vi "Laser 1 Operations L3.vi"(8 "Error in":errorcluster caption="Error in (no error)", 11 "UI elements cluster":T2) -> (0 "Error out":errorcluster)   [LabVIEW 2020]
uses:
  Typedefs/UI ctrl refs cluster.ctl
  Typedefs/Laser control knob.ctl
  Typedefs/Frame Size.ctl
  Typedefs/Plane Mode.ctl
  Typedefs/PMT control knob.ctl
  Typedefs/XY Stage_Move.ctl
  Typedefs/test_fpga_control.ctl
  Acquisition/Typedefs/Ref DAQ Param.ctl
  User Interface/Misc/Experiment Type.ctl
  User Interface/Misc/Biology Information.ctl
  Type Defs/Ls1 Operations.ctl
  Typedefs/HW config states enum.ctl
  Type Defs/Ls1 User Ops.ctl
  Serial Comms/Visa resource.ctl
  Typedefs/fgv_actions.ctl
  Global Variables/General Globals.vi
  Global Variables/gl_UI Ctrl Refs.vi
panel:
  out "Laser Ops  actions":T1
  out "Loop itr":i32
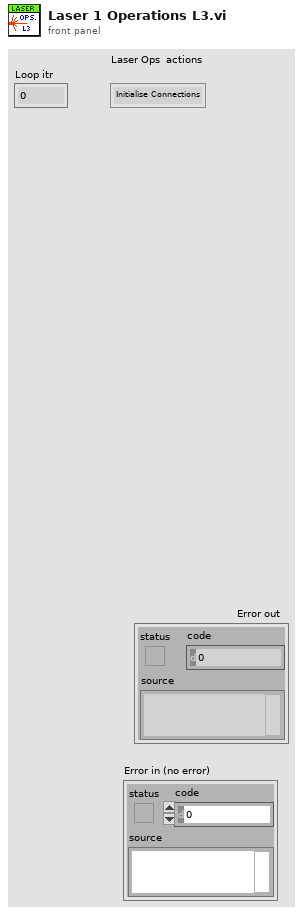
[diagram p1: front panel]
types:
  T1 = typedef "Ls1 Operations.ctl" = enum16{"Initialise Connections", "Initialise system", "Check Status", "Open/Close Shutter", "Start/Stop Pump Peak Hold", "Set wavelength", "Close"}
  T2 = typedef "UI ctrl refs cluster.ctl" = cluster{"Top level VI path":path, "Top level VI ref":refnum<vi>, "User menu ref":refnum<k9>, "Sub Panel control":refnum<vi>, "Imaging Param Tab":refnum<vi>, "Occurrence-Start drivers":refnum<k4>, "Occurrence-Speed logging initialised":refnum<k4>, "Occurrence-XYZ stage initialised":refnum<k4>, "Exit button":refnum<vi>, "Status ind":refnum<vi>, "Set as origin":refnum<vi>, "Speed Logging":refnum<vi>, "Time Lapse":refnum<vi>, "Live Imaging":refnum<vi>, "AOL Z Stack":refnum<vi>, "Motor Z Stack":refnum<vi>, "Funct Acq button":refnum<vi>, "Hard Shutter":refnum<vi>, "Virtual Shutter":refnum<vi>, "Laser Power":refnum<vi>, "AOL Mode":refnum<vi>, "Frame Size":refnum<vi>, "Field of View":refnum<vi>, "Dwell Time":refnum<vi>, "Zoom":refnum<vi>, "AOL Z":refnum<vi>, "Objective":refnum<vi>, "Axis":refnum<vi>, "Paths & Names":refnum<vi>, "Experiment folder path (ind.)":refnum<vi>, "Last State (Ind.)":refnum<vi>, "Averages":refnum<vi>, "Angle (degrees)":refnum<vi>, "X centre":refnum<vi>, "Y centre":refnum<vi>, "Plane Mode":refnum<vi>, "# Planes":refnum<vi>, "Z Start":refnum<vi>, "Z Stop":refnum<vi>, "Z Step":refnum<vi>, "PMT 1":refnum<vi>, "PMT 2":refnum<vi>, "Stage XYZ Position":refnum<vi>, "Pockels@Z Start":refnum<vi>, "Pockels@Z Stop":refnum<vi>, "Obtain Z Start":refnum<vi>, "Obtain Z Stop":refnum<vi>, "Live stim.trig.period":refnum<vi>, "Live stim.trig.enable":refnum<vi>, "Movement Correction":refnum<vi>, "Load Reference Image":refnum<vi>, "XY Stage Move":refnum<vi>, "MovCor Cluster":refnum<vi>, "RefDAQParam":refnum<vi>, "Funct. Acq. Pockels Modulation":refnum<vi>, "Ref Laser Power":refnum<vi>, "Enable Video Recording":refnum<vi>, "Video Record-Live Imaging":refnum<vi>, "Video Record-Funct acq":refnum<vi>, "Reference Source":refnum<vi>, "AOL Z-stack Chirps Ready (ind)":refnum<vi>, "Target time between mov.cor. ref triggers (ms)":refnum<vi>, "Funct. Acq. Ref frame save":refnum<vi>, "Tracking button":refnum<vi>, "Show ref plots window":refnum<vi>, "Center freq ind (nm)":refnum<vi>, "Pickup mode (ind)":refnum<vi>, "Logging queue (ind)":refnum<vi>, "Back aperture power (ind.)":refnum<vi>, "Power after objective (ind.)":refnum<vi>, "Switch user":refnum<vi>, "Ls1 Conn. Status":refnum<vi>, "Ls1Tuning Status":refnum<vi>, "Ls1 Faults":refnum<vi>, "Ls1 Connection":refnum<vi>, "Ls1 Mode":refnum<vi>, "Ls1 POWER [mW]":refnum<vi>, "Ls1Shutter":refnum<vi>, "Ls1 Wavelength":refnum<vi>, "Ls1 Note":refnum<vi>, "Ls1 Confirm Wav":refnum<vi>, "Ls1 PreChrp Prism1":refnum<vi>, "Ls1 PreChrp Prism2":refnum<vi>, "Ls1 wav top Ind":refnum<vi>, "Ls1 power top Ind":refnum<vi>, "Ls1 Pump peak Hold":refnum<vi>, "Ls1 Status Ind":refnum<vi>, "Ls1 wav cancel":refnum<vi>, "Experiment Type":refnum<vi>, "Biology Information":refnum<vi>, "Camera recording status":refnum<vi>, "Optimise Obj. Pos.":refnum<vi>}
  T3 = typedef "Ls1 User Ops.ctl" = enum16{"Setup", "Initialise", "Disable Controls", "Enable Controls", "Update Connection Info", "Update Laser Warning", "Update Laser status", "Update Laser status - sel", "Update Laser Wav.", "Update Laser Power", "Update prechiper settings", "Update Laser Note", "Update Shutter Status", "Close"}
  T4 = typedef "HW config states enum.ctl" = enum16{"Load from file", "Save to file", "Save backup", "Write all", "Read all", "Write XY stage settings", "Write DAQ FPGA settings", "Write Control FPGA settings", "Write Phys Channels", "Write System Config", "Write HW Config", "Save System Config", "Save HW Config", "Clear", "Compare from file"}
  T5 = typedef "Visa resource.ctl" = cluster{"VISA resource name":refnum<visa-resource-name>, "baud rate":u32}
  T6 = typedef "fgv_actions.ctl" = enum16{"Get", "Set"}
  T7 = typedef "System Configuration.ctl" = cluster{"Laser wavelength (nm)":dbl, "DAQ FPGA System":T8, "Control system":T9}
  T8 = typedef "DAQ FPGA system config.ctl" = cluster{"Clock Freq (MHz) ":dbl, "Samples Wait after Trigger":u16, "AOD fill":u16, "StartupDelay":i32, "Slip Cycle (clock cycles)":u32, "Add Cycle":bool}
  T9 = typedef "CTRL system config.ctl" = cluster{"AOD 1 Amplitude":i16, "AOD 2 Amplitude":i16, "AOD 3 Amplitude":i16, "AOD 4 Amplitude":i16, "AOD 5 Amplitude":i16, "AOD 6 Amplitude":i16, "T0 (ns)":dbl, "Ta (ns)":dbl, "Data Time Interval (ns)":dbl, "Ctrl FPGA Clock (MHz)":dbl}
  T10 = typedef "Hardware Configuration settings.ctl" = cluster{"Dev. PC":bool, "Swap XY on stage":bool, "No of AOD":u8, "MC Supported":bool, "Axial MC":bool, "Computer MAC address":string, "Externalise Triggers":bool, "Trigger HW config":T11, "DAQmx Chan":T12, "XYZ Stage Control Config":T13, "XY stage available":bool, "XY Comms Config Cluster":T14, "Y stage available":bool, "Y Comms Config Cluster":T14, "Z stage available":bool, "Z Comms Config Cluster ":T14, "Encoder available":bool, "Encoder":T16, "VidRec available":bool, "Cam VidRec":T17, "Laser Power Control HW config":T18, "Laser 1 available":bool, "Laser 1 config cluster":T19, "Prechirper 1 available":bool, "Prechirper 1 config cluster":T20, "Control system.FPGA available?":bool, "Control Sys. HW config":T21, "DAQ FPGA HW Config":T22, "PMT Control Voltage Limits":T26}
  T11 = typedef "Triggers HW config.ctl" = cluster{"Available Device List":i32, "Device Address":string}
  T12 = typedef "DAQmx physical channels cluster.ctl" = cluster{"Pockels AO":tag, "Hard shutter AO":tag, "PMT AOs":tag, "Galvo AOs":tag, "Power meter AI":tag}
  T13 = typedef "XYZControlConfig.ctl" = enum16{"None", "XYZ", "XY-Z", "X-Y-Z", "Z"}
  T14 = typedef "Peripherals comms config cluster.ctl" = cluster{"Name":string, "Device Address":string, "Port ":u16, "Baudrate":i32, "Comms Type":T15}
  T15 = typedef "Comms Type.ctl" = enum16{"GPIB-IEEE488", "Serial-RS232", "Serial-RS485", "Serial-RS422", "Serial-USB", "Ethernet-TCP/IP", "Ethernet-UDP"}
  T16 = typedef "Encoder config cluster.ctl" = cluster{"IP address":string, "Port":u16, "Wheel radius (cm)":dbl, "Encoder Trigger":tag}
  T17 = typedef "Cam VidRec HW config setup cluster.ctl" = cluster{"DO flag-Video record":tag, "DO flag-Trial start":tag}
  T18 = typedef "Laser Power Control HW config.ctl" = cluster{"Laser Power Control":string, "Laser Power Modulation Control":enum16{"NI", "FPGA"}}
  T19 = typedef "Laser 1 config cluster.ctl" = cluster{"COM port":refnum<visa-resource-name>, "Baud Rate":i32, "Type":string}
  T20 = typedef "PreChirper 1 config cluster.ctl" = cluster{"Type":string, "Baud Rate":i32, "COM port":refnum<visa-resource-name>}
  T21 = typedef "Control Sys HW config cluster.ctl" = cluster{"Control system.FPGA Type":enum16{"Virtex 5", "Virtex 7"}, "Control system.Network adapter name":string, "Control system.MAC address":string, "Control system.Ethernet Port":u32, "Control system.Ethernet Port Opened":bool}
  T22 = typedef "DAQ FPGA HW config cluster.ctl" = cluster{"FGPA Ref":T23, "Target":T24, "input card type":T25}
  T23 = typedef "FPGA Ref.ctl" = refnum<k20>
  T24 = typedef "nirio_resource_hc.ctl" = tag
  T25 = typedef "FPGA input type AC-DC.ctl" = enum16{"AC Card", "DC Card"}
  T26 = typedef "PMT Control Voltage limits.ctl" = cluster{"Lower Limit":dbl, "Upper Limit":dbl}
  T27 = typedef "AOL_Globals.ctl" = cluster{"Imaging Protocol":T28, "Number of POI":u16, "Number of Miniscans":u16, "Number of Trials":u16, "Number of Cycles ":u64, "# Averaged Frames":u16, "Laser power (%)":u8, "Pockels (V)":dbl, "Acquisition Length (sec)":dbl, "Fill time (us)":dbl, "POI Dwell time (us)":dbl, "Miniscan Dwell time per pixel (us)":dbl, "PMT 1":dbl, "PMT 2":dbl, "Back Apperture (mA)":dbl, "Frame Size":T29, "Center Frequency":dbl, "Field of View (um)":dbl, "Field of View (norm)":dbl, "DwellTime (us)":dbl, "Ref Dwell Time (us)":dbl, "Wavelength (nm)":dbl, "Zoom":dbl, "AOL Z":dbl, "AOL Mode":T30, "GridXY":dbl, "GridZ":dbl, "TriggerPeriod (sec)":dbl, "Number of Pixels in Miniscan":u16, "Experiment folder path":path, "X centre":dbl, "Y centre":dbl, "Angle (degrees)":dbl, "Angle Xs (degrees)":dbl, "Angle Ys (degrees)":dbl, "Plane Mode":T31, "Threshold":u16[], "Regenerate Chirps":bool, "Rectangle ROI length (pixels)":u16, "Rectangle ROI height (pixels)":u16, "AOD fill":u16, "StartupDelay":i32, "Samples Wait after Trigger":u16, "Slip Cycle":u32, "Add Cycle":bool, "Functional Mode":T32, "Z Start":dbl, "Z Stop":dbl, "# Planes":i32, "Total Pixels":i32, "Variable Miniscan Pixels":u16[], "Use Variable Length":bool, "Use Variable Resolution":bool, "Laser power (%) at Z Start":u8, "Laser power (%) at Z Stop":u8, "Ref Z Step":i8}
  T28 = typedef "Imaging Protocols enum.ctl" = enum16{"AOL Z-Stack", "Motor Z Stack", "Parameter Sweep", "Functional Acquisition", "Single Plane Acquisition", "Volume Acquisition", "Live Imaging", "Live Plane Imaging", "Live Volume Imaging"}
  T29 = typedef "Frame Size.ctl" = u16
  T30 = typedef "AOL modes.ctl" = enum16{"Raster", "Structural", "Pointing", "Mini Scan", "Alignment"}
  T31 = typedef "Plane Mode.ctl" = u16
  T32 = typedef "Functional Mode.ctl" = enum16{"Point", "Line", "Patch", "Plane", "Volume"}
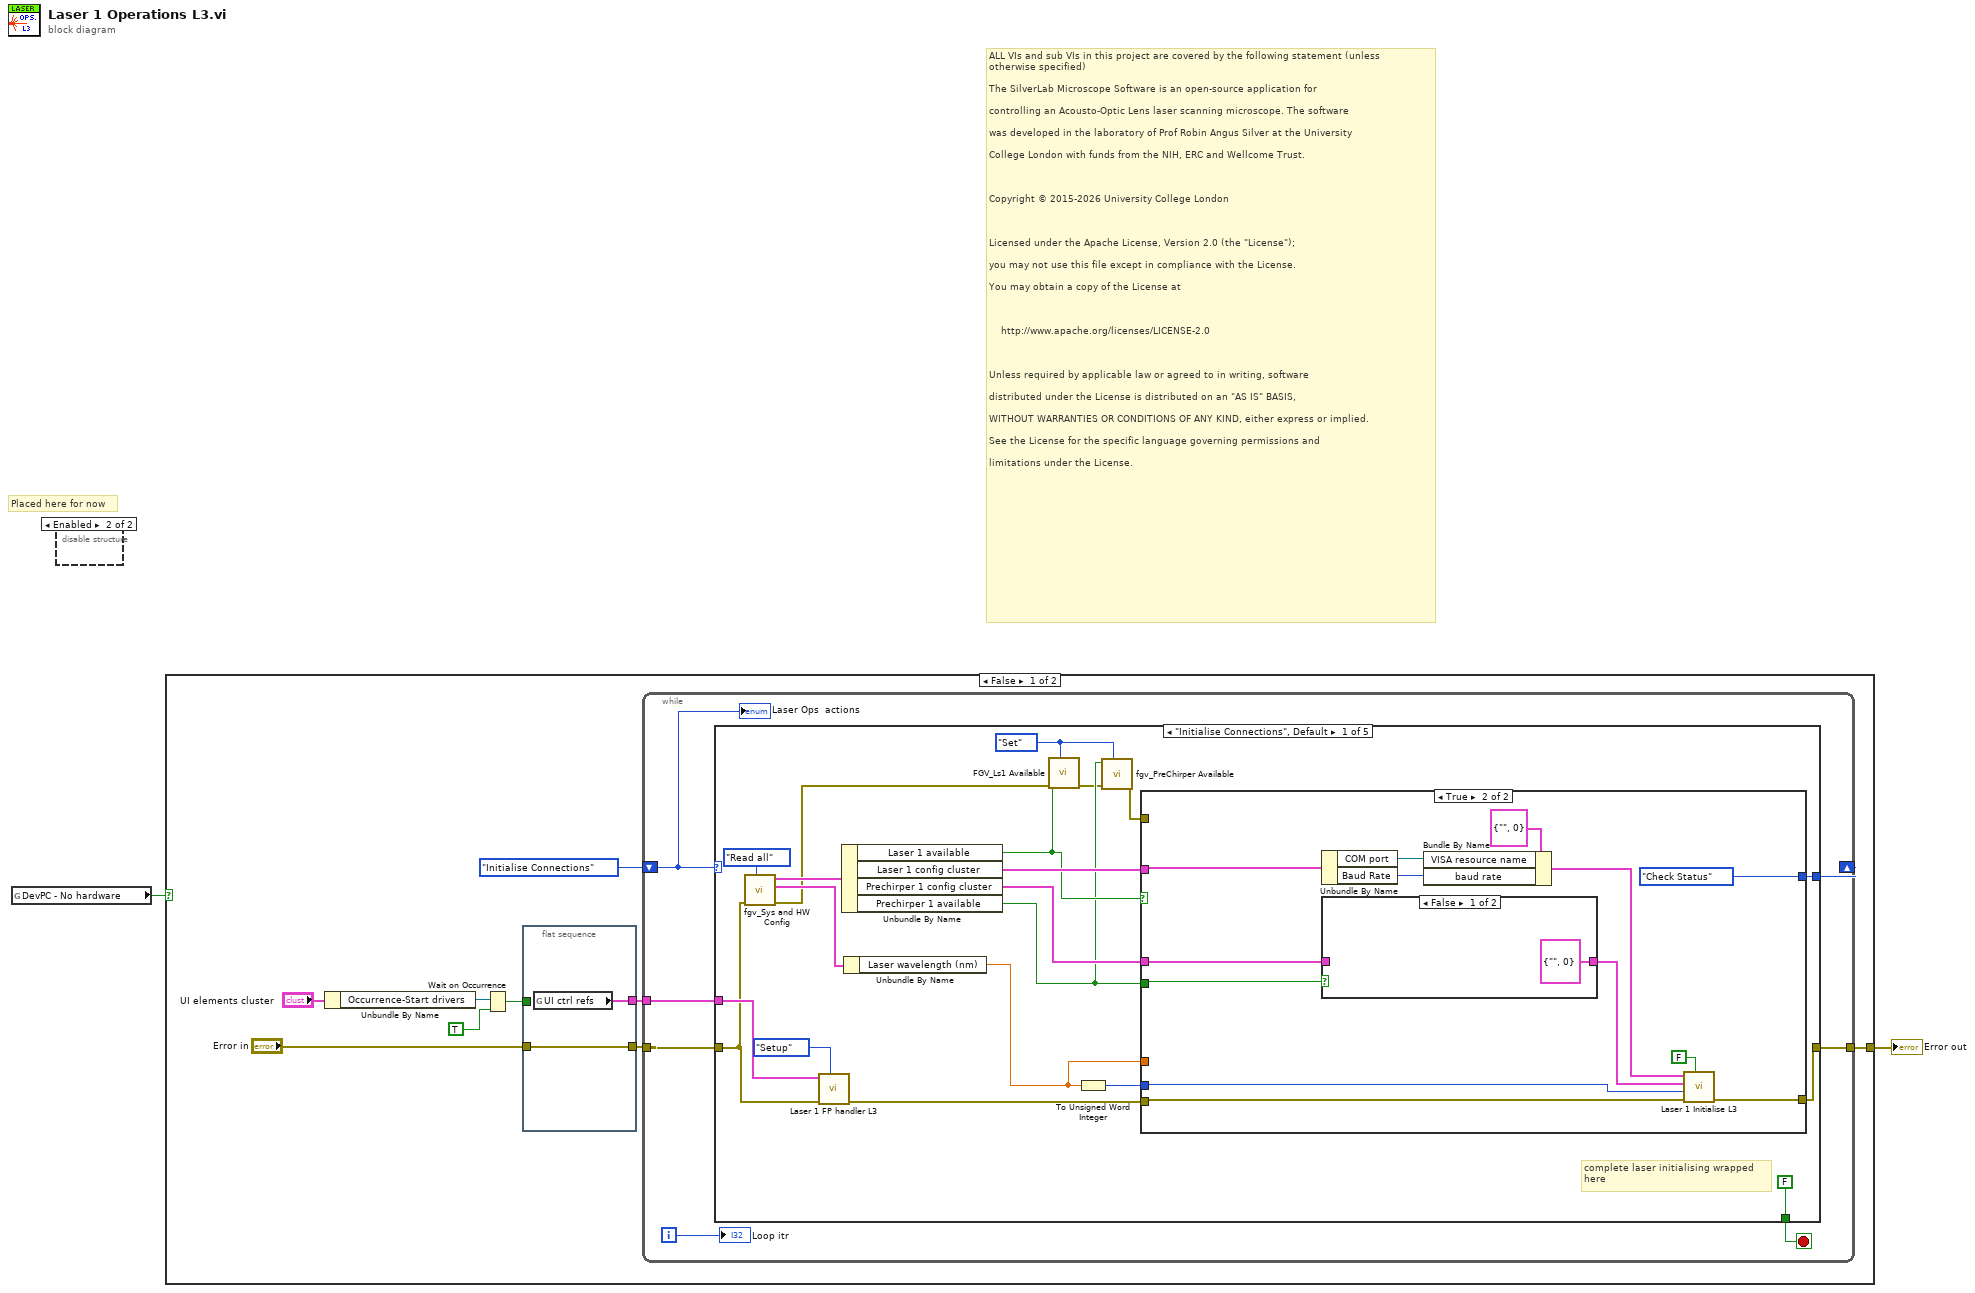
[diagram p0: block diagram]
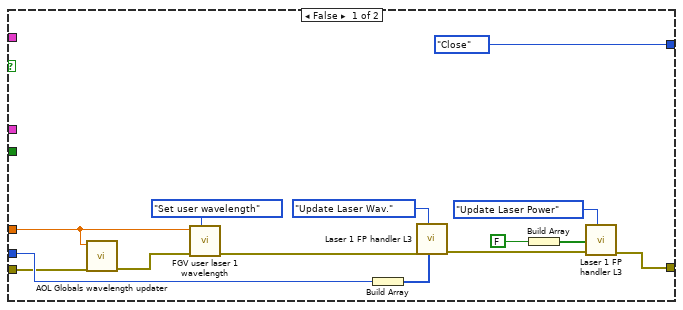
[diagram p2: hidden frame]
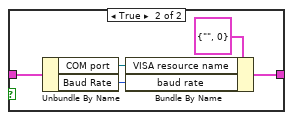
[diagram p3: hidden frame]
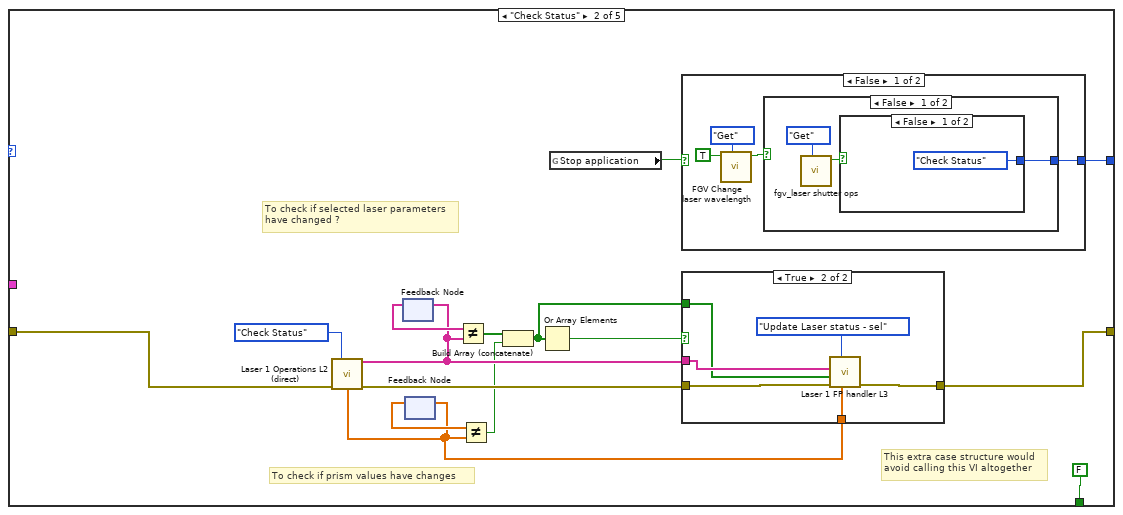
[diagram p4: hidden frame]
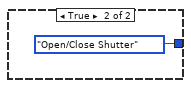
[diagram p5: hidden frame]
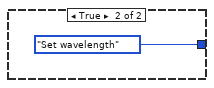
[diagram p6: hidden frame]
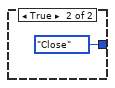
[diagram p7: hidden frame]
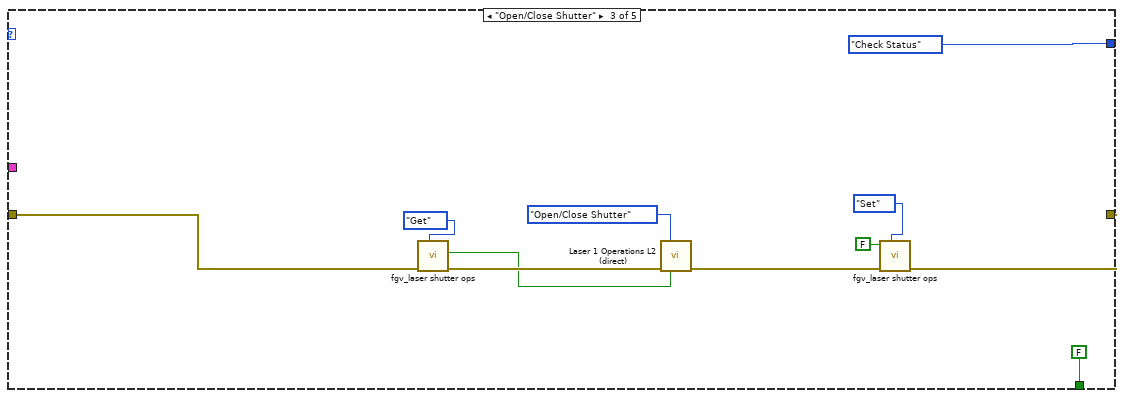
[diagram p9: hidden frame]
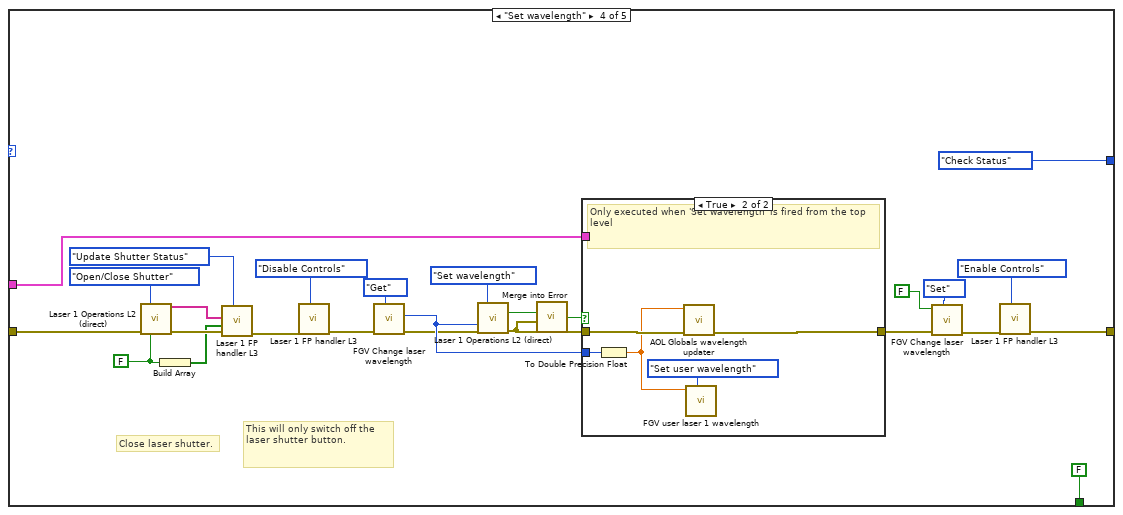
[diagram p10: hidden frame]
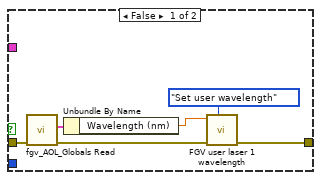
[diagram p11: hidden frame]
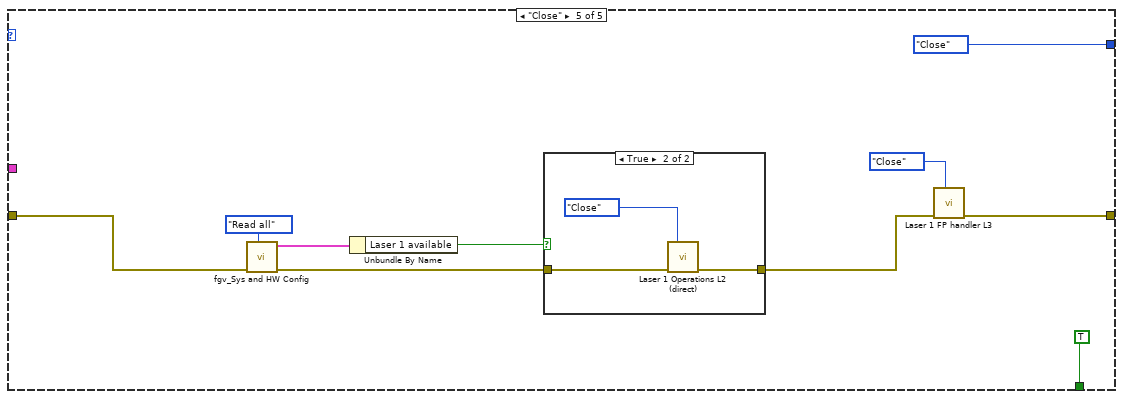
[diagram p12: hidden frame]
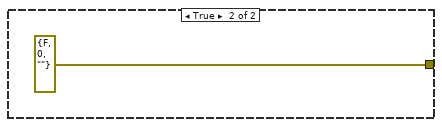
[diagram p14: hidden frame]
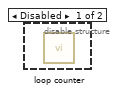
[diagram p15: hidden frame]
diagram:
  # "ALL VIs and sub VIs in this project are covered by the following statement (unless \notherwise specified)\n\nThe SilverLab Microscope Software is an open-source application for\n\ncontrolling an Acousto-Optic Lens laser scanning microscope. The software\n\nwas developed in the laboratory of Prof Robin Angus Silver at the University\n\nCollege London with funds from the NIH, ERC and Wellcome Trust.\n\n \n\nCopyright © 2015-2026 University College London\n\n \n\nLicensed under the Apache License, Version 2.0 (the \"License\");\n\nyou may not use this file except in compliance with the License.\n\nYou may obtain a copy of the License at\n\n \n\n    http://www.apache.org/licenses/LICENSE-2.0\n\n \n\nUnless required by applicable law or agreed to in writing, software\n\ndistributed under the License is distributed on an \"AS IS\" BASIS,\n\nWITHOUT WARRANTIES OR CONDITIONS OF ANY KIND, either express or implied.\n\nSee the License for the specific language governing permissions and\n\nlimitations under the License."
  # "Placed here for now"
  n1 = global read "General Globals.vi" "DevPC - No hardware"() -> (w1:bool)
  n2 = disable-structure shown="Enabled" {
    frame Disabled {
      n3 = call "loop counter.vi"() -> ()  [unwired: 9 in, 1 out]
    }
    frame Enabled {
    }
  }
  n4 = case shown="False" w1 {
    tunnel: [w11 errorcluster {"status"=FALSE, "code"=0, "source"=""} ("error out")] -> w2
    frame False {
      n5 = Unbundle By Name("UI elements cluster") -> ("Occurrence-Start drivers"=w6:refnum<k4>)
      n6 = Wait on Occurrence(1:TRUE ("ignore previous (T)"), 2:w6) -> (0:w5:bool)  [unwired: 1 in]
      n7 = flat-sequence {
        tunnel: w5 -> [_]
        tunnel: "Error in" -> [w13]
        tunnel: [w13] -> w9
        tunnel: [w12] -> w3
        frame #0 {
          n8 = global read "gl_UI Ctrl Refs.vi" "UI ctrl refs"() -> (w12:T2)
        }
      }
      n9 = while {
        tunnel: w9 -> [w20]
        tunnel: w3 -> [w19]
        shift-right: [w16] -> _
        shift-left: Ls1_Operations."Initialise Connections" ("Laser Ops\n actions") -> [w17]
        tunnel: [w18] -> w11
        i -> [w14]
        stop <- w15 stop-if-true
        n10 = case shown="\"Initialise Connections\", Default" w17 {
          tunnel: w20 -> [w24 w88 w113 w130 w161]
          tunnel: w19 -> [w40 _ _ w139 _]
          tunnel: [w39 w83 w107 w119 w155] -> w18
          tunnel: [w34 w81 Ls1_Operations."Check Status" ("Laser Ops\n actions") Ls1_Operations."Check Status" ("Laser Ops\n actions") Ls1_Operations."Close" ("Laser Ops\n actions")] -> w16
          tunnel: [FALSE FALSE FALSE FALSE TRUE] -> w15
          frame "Initialise Connections", Default {
            w30 = enum16{"Get", "Set"}."Set" ("FGV Actions")
            # "complete laser initialising wrapped \nhere"
            n11 = call "fgv_Sys and HW Config.vi"("Function"=HW_config_states_enum."Read all", "error in (no error)"=w24) -> ("error out"=w23:errorcluster, "System Config OUT"=w27:T7, "Hardware Configuration OUT"=w28:T10)  [unwired: 7 in]
            n12 = call "Laser 1 FP handler L3.vi"("FP Ops"=Ls1_User_Ops."Setup", "Error in"=w24, "UI elements cluster"=w40) -> ("Error out"=w26:errorcluster)  [unwired: 6 in, 2 out]
            n13 = Unbundle By Name(w28) -> ("Laser 1 available"=w31:bool, "Laser 1 config cluster"=w38:T19, "Prechirper 1 config cluster"=w37:T20, "Prechirper 1 available"=w29:bool)
            n14 = Unbundle By Name(w27) -> ("Laser wavelength (nm)"=w25:dbl)
            n15 = call "FGV_Ls1 Available.vi"("FGV Actions"=w30, "error in (no error)"=w23, "Laser Available ? IN"=w31) -> ("error out"=w22:errorcluster)  [unwired: 7 in, 1 out]
            n16 = To Unsigned Word Integer(number=w25) -> (unsigned 16bit integer=w35:u16)
            n17 = call "fgv_PreChirper Available.vi"("FGV Actions"=w30, "error in (no error)"=w22, "PreChirper Available ? IN"=w29) -> ("error out"=w21:errorcluster)  [unwired: 7 in, 1 out]
            n18 = case shown="True" w31 {
              tunnel: [w44 w67] -> w39
              tunnel: w38 -> [_ w63]
              tunnel: w37 -> [_ w62]
              tunnel: w26 -> [w43 w61]
              tunnel: w35 -> [w52 w60]
              tunnel: [Ls1_Operations."Close" ("Laser Ops\n actions") Ls1_Operations."Check Status" ("Laser Ops\n actions")] -> w34
              tunnel: w25 -> [w41 _]
              tunnel: w29 -> [_ w55]
              tunnel: w21 -> [_ _]
              frame False {
                n19 = call "AOL Globals wavelength updater.vi"("error in (no error)"=w43, "Laser wavelength (nm)"=w41) -> ("error out"=w42:errorcluster)  [unwired: 9 in]
                n20 = call "FGV user laser 1 wavelength.vi"("FGV Actions"=enum16{"Get", "Set user wavelength"}."Set user wavelength", "error in (no error)"=w42, "Laser wavelength IN"=w41) -> ("error out"=w45:errorcluster)  [unwired: 7 in, 1 out]
                n21 = Build Array(w52) -> (w51:u16[])
                n22 = call "Laser 1 FP handler L3.vi"("Numeric"=w51, "FP Ops"=Ls1_User_Ops."Update Laser Wav.", "Error in"=w45) -> ("Error out"=w50:errorcluster)  [unwired: 6 in, 2 out]
                n23 = Build Array(FALSE) -> (w47:bool[])
                n24 = call "Laser 1 FP handler L3.vi"("FP Ops"=Ls1_User_Ops."Update Laser Power", "Error in"=w50, "Boolean"=w47) -> ("Error out"=w44:errorcluster)  [unwired: 6 in, 2 out]
              }
              frame True {
                n25 = Unbundle By Name(w63) -> ("COM port"=w58:refnum<visa-resource-name>, "Baud Rate"=w57:i32)
                n26 = case shown="False" w55 {
                  tunnel: [T5 {"VISA resource name"="", "baud rate"=0} ("Ls1 Visa \nresource") w73] -> w64
                  tunnel: w62 -> [_ w72]
                  frame False {
                  }
                  frame True {
                    n27 = Unbundle By Name(w72) -> ("COM port"=w70:refnum<visa-resource-name>, "Baud Rate"=w69:i32)
                    n28 = Bundle By Name(cluster=T5 {"VISA resource name"="", "baud rate"=0} ("Ls1 Visa \nresource"), "VISA resource name"=w70, "baud rate"=w69) -> (w73:T5)
                  }
                }
                n29 = Bundle By Name(cluster=T5 {"VISA resource name"="", "baud rate"=0} ("Ls1 Visa \nresource"), "VISA resource name"=w58, "baud rate"=w57) -> (w65:T5)
                n30 = call "Laser 1 Initialise L3.vi"("Independent?"=FALSE ("from FGV ?"), "Error in"=w61, "Wavelength (set) [nm]"=w60, "PreChrp1 \nVisa resource"=w64, "Ls1 Visa \nresource"=w65) -> ("Error out"=w67:errorcluster)  [unwired: 6 in]
              }
            }
          }
          frame "Check Status" {
            # "This extra case structure would\navoid calling this VI altogether"
            # "To check if prism values have changes"
            # "To check if selected laser parameters\nhave changed ?"
            n31 = call "Laser 1 Operations L2 (direct).vi"("Laser Ops\n actions"=Ls1_Operations."Check Status" ("Laser Ops\n actions"), "error in (no error)"=w88) -> ("Ls Data"=w82:string[], "prism Values"=w74:dbl[], "error out"=w84:errorcluster)  [unwired: 8 in, 3 out]
            n32 = feedback-in #1(w82) -> ()
            n33 = feedback #1() -> (w85:string[])  [unwired: 1 in]
            n34 = feedback #2() -> (w78:dbl[])  [unwired: 1 in]
            n35 = feedback-in #2(w74) -> ()
            n36 = Not Equal?(x=w85, y=w82) -> (x != y?=w77:bool[])
            n37 = Not Equal?(x=w78, y=w74) -> (x != y?=w76:bool)
            n38 = Build Array (concatenate)(w77, w76) -> (w75:bool[])
            n39 = Or Array Elements(Boolean array=w75) -> (logical OR=w79:bool)
            n40 = global read "General Globals.vi" "Stop application"() -> (w80:bool)
            n41 = case shown="False" w80 {
              tunnel: [w89 Ls1_Operations."Close" ("Laser Ops\n actions")] -> w81
              frame False {
                n42 = call "FGV Change laser wavelength.vi"("FGV Actions"=enum16{"Get", "Set"}."Get", "Change Wavelength ? IN"=TRUE) -> ("Change Wavelength ? OUT"=w90:bool)  [unwired: 7 in, 2 out]
                n43 = case shown="False" w90 {
                  tunnel: [w93 Ls1_Operations."Set wavelength" ("Laser Ops\n actions")] -> w89
                  frame False {
                    n44 = call "fgv_laser shutter ops.vi"("FGV Actions"=fgv_actions."Get") -> ("Operate Shutter [OUT}"=w94:bool)  [unwired: 8 in, 2 out]
                    n45 = case shown="False" w94 {
                      tunnel: [Ls1_Operations."Check Status" ("Laser Ops\n actions") Ls1_Operations."Open/Close Shutter" ("Laser Ops\n actions")] -> w93
                      frame False {
                      }
                      frame True {
                      }
                    }
                  }
                  frame True {
                  }
                }
              }
              frame True {
              }
            }
            n46 = case shown="True" w79 {
              tunnel: w84 -> [w100 w106]
              tunnel: [w100 w105] -> w83
              tunnel: w82 -> [_ w103]
              tunnel: w75 -> [_ w102]
              tunnel: w74 -> [_ w101]
              frame False {
              }
              frame True {
                n47 = call "Laser 1 FP handler L3.vi"("Numeric"=w101, "FP Ops"=Ls1_User_Ops."Update Laser status - sel", "Error in"=w106, "Boolean"=w102, "I/p string(s)"=w103) -> ("Error out"=w105:errorcluster)  [unwired: 4 in, 2 out]
              }
            }
          }
          frame "Open/Close Shutter" {
            n48 = call "fgv_laser shutter ops.vi"("FGV Actions"=fgv_actions."Get", "error in (no error)"=w113) -> ("error out"=w112:errorcluster, "Shutter state [OUT]"=w111:bool)  [unwired: 7 in, 1 out]
            n49 = call "Laser 1 Operations L2 (direct).vi"("Laser Ops\n actions"=Ls1_Operations."Open/Close Shutter" ("Laser Ops\n actions"), "error in (no error)"=w112, "Boolean I/P"=w111) -> ("error out"=w108:errorcluster)  [unwired: 7 in, 5 out]
            n50 = call "fgv_laser shutter ops.vi"("FGV Actions"=fgv_actions."Set", "error in (no error)"=w108, "Operate Shutter"=FALSE) -> ("error out"=w107:errorcluster)  [unwired: 6 in, 2 out]
          }
          frame "Set wavelength" {
            w126 = FALSE ("Boolean I/P")
            # "This will only switch off the \nlaser shutter button."
            # "Close laser shutter."
            n51 = call "Laser 1 Operations L2 (direct).vi"("Laser Ops\n actions"=Ls1_Operations."Open/Close Shutter" ("Laser Ops\n actions"), "error in (no error)"=w130, "Boolean I/P"=w126) -> ("Ls Data"=w118:string[], "error out"=w128:errorcluster)  [unwired: 7 in, 4 out]
            n52 = Build Array(w126) -> (w125:bool[])
            n53 = call "Laser 1 FP handler L3.vi"("FP Ops"=Ls1_User_Ops."Update Shutter Status", "Error in"=w128, "Boolean"=w125, "I/p string(s)"=w118) -> ("Error out"=w123:errorcluster)  [unwired: 5 in, 2 out]
            n54 = call "Laser 1 FP handler L3.vi"("FP Ops"=Ls1_User_Ops."Disable Controls", "Error in"=w123) -> ("Error out"=w122:errorcluster)  [unwired: 7 in, 2 out]
            n55 = call "FGV Change laser wavelength.vi"("FGV Actions"=enum16{"Get", "Set"}."Get", "error in (no error)"=w122) -> ("error out"=w131:errorcluster, "Wavelength OUT"=w132:i16)  [unwired: 7 in, 1 out]
            n56 = call "Laser 1 Operations L2 (direct).vi"("Laser Ops\n actions"=Ls1_Operations."Set wavelength" ("Laser Ops\n actions"), "Wavelength \n(set) [nm]"=w132, "error in (no error)"=w131) -> ("Resp Validated"=w143:bool, "error out"=w142:errorcluster)  [unwired: 7 in, 4 out]
            n57 = call "Merge into Error.vi"("Boolean in"=w143, "error in (no error)"=w142) -> ("Boolean out"=w141:bool)  [unwired: 6 in]
            n58 = case shown="True" w141 {
              tunnel: w142 -> [w147 w152]
              tunnel: [w145 w151] -> w134
              tunnel: w132 -> [_ w154]
              tunnel: w139 -> [_ _]
              frame False {
                n59 = call "fgv_AOL_Globals Read.vi"("error in (no error)"=w147) -> ("error out"=w146:errorcluster, "AOL_Globals"=w149:T27)  [unwired: 8 in, 1 out]
                n60 = Unbundle By Name(w149) -> ("Wavelength (nm)"=w144:dbl)
                n61 = call "FGV user laser 1 wavelength.vi"("FGV Actions"=enum16{"Get", "Set user wavelength"}."Set user wavelength", "error in (no error)"=w146, "Laser wavelength IN"=w144) -> ("error out"=w145:errorcluster)  [unwired: 7 in, 1 out]
              }
              frame True {
                # "Only executed when 'Set wavelength' is fired from the top level"
                n62 = To Double Precision Float(number=w154) -> (double precision float=w150:dbl)
                n63 = call "AOL Globals wavelength updater.vi"("error in (no error)"=w152, "Laser wavelength (nm)"=w150) -> ("error out"=w151:errorcluster)  [unwired: 9 in]
                n64 = call "FGV user laser 1 wavelength.vi"("FGV Actions"=enum16{"Get", "Set user wavelength"}."Set user wavelength", "Laser wavelength IN"=w150) -> ()  [unwired: 8 in, 2 out]
              }
            }
            n65 = call "FGV Change laser wavelength.vi"("FGV Actions"=enum16{"Get", "Set"}."Set", "error in (no error)"=w134, "Change Wavelength ? IN"=FALSE) -> ("error out"=w120:errorcluster)  [unwired: 6 in, 2 out]
            n66 = call "Laser 1 FP handler L3.vi"("FP Ops"=Ls1_User_Ops."Enable Controls", "Error in"=w120) -> ("Error out"=w119:errorcluster)  [unwired: 7 in, 2 out]
          }
          frame "Close" {
            n67 = call "fgv_Sys and HW Config.vi"("Function"=HW_config_states_enum."Read all", "error in (no error)"=w161) -> ("error out"=w160:errorcluster, "Hardware Configuration OUT"=w159:T10)  [unwired: 7 in, 1 out]
            n68 = Unbundle By Name(w159) -> ("Laser 1 available"=w158:bool)
            n69 = case shown="True" w158 {
              tunnel: [w165 w168] -> w156
              tunnel: w160 -> [w165 w166]
              frame False {
              }
              frame True {
                n70 = call "Laser 1 Operations L2 (direct).vi"("Laser Ops\n actions"=Ls1_Operations."Close" ("Laser Ops\n actions"), "error in (no error)"=w166) -> ("error out"=w168:errorcluster)  [unwired: 8 in, 5 out]
              }
            }
            n71 = call "Laser 1 FP handler L3.vi"("FP Ops"=Ls1_User_Ops."Close", "Error in"=w156) -> ("Error out"=w155:errorcluster)  [unwired: 7 in, 2 out]
          }
        }
        "Loop itr" <- w14
        "Laser Ops  actions" <- w17
      }
    }
    frame True {
    }
  }
  "Error out" <- w2
